vi "Intake Controller.vi"(8 "error in":errorcluster) -> ()   [LabVIEW 2017]
doc: "This VI executes continuously carrying out the current operation and responding to updates or new operations. It will often contain the timing or control code that is difficult to place directly in TeleOp. This VI generally opens all sensors and motors and isolates the rest of the robot code from knowing how the operations are carried out."
uses:
  <vilib>/Rock Robotics/WPI/Framework/Completion Status.ctl
  Intake Setpoints.ctl
  Intake Operations.ctl
  <vilib>/Rock Robotics/SystemInterfaces/DIO/FPGA_DIOPWMChannel.ctl
  <vilib>/Rock Robotics/WPI/RobotDrive/WPI_RobotDriveOpen2MotorWithSPARK.vi
  <vilib>/Rock Robotics/Network Tables/NT Write Boolean.vi
  Framework/Robot Global Data.vi
panel:
  in  "Interactive Values":T1
  out "Current\nCmd":string="Started at  12:56:38.436\nDefault: Reserve,  S 0.0, D 0.000000"
  in  "Buttons":cluster{"Execute Cmd":bool, "Abort Cmd":bool}
  out "Command Timing":cluster{"Start Time (ms)":u32, "Iterations":i32}={"Start Time (ms)"=8116528, "Iterations"=0}
  out "Status":T3
  # "Tip: It may be helpful to observe inputs and sensor values.\nYou may also want to display tuning or debugging controls."
  # "Interactive Command: You may fill in the settings for a command\nand schedule it with the Execute button. You can observe and abort\nany command while fine tuning the code for the controller."
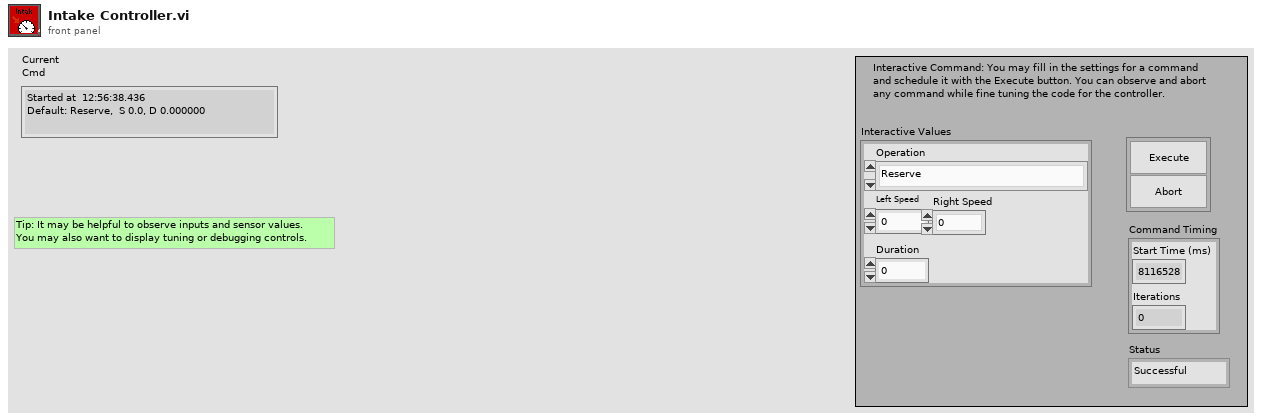
[diagram p1: front panel]
types:
  T1 = typedef "Intake Setpoints.ctl" = cluster{"Operation":T2, "Left Speed":dbl, "Duration":dbl, "Right Speed":dbl}
  T2 = typedef "Intake Operations.ctl" = enum16{"Reserve", "Read Current", "Immediate", "Intake for Duration", "Intake Until Cube"}
  T3 = typedef "Completion Status.ctl" = enum16{"Successful", "Aborted", "Incomplete"}
  T4 = typedef "FPGA_DIOPWMChannel.ctl" = enum8{"PWM 0", "PWM 1", "PWM 2", "PWM 3", "PWM 4", "PWM 5", "PWM 6", "PWM 7", "PWM 8", "PWM 9", "PWM MXP 0", "PWM MXP 1", "PWM MXP 2", "PWM MXP 3", "PWM MXP 4", "PWM MXP 5", "PWM MXP 6", "PWM MXP 7", "PWM MXP 8", "PWM MXP 9", "Invalid"}
  T5 = typedef "WPI_RobotDriveDevRef.ctl" = cluster{"DevStatus":errorcluster, "Motors[]":T6[], "Square Inputs":bool, "Max Output":dbl}
  T6 = typedef "WPI_MotorControlDeviceRef.ctl" = cluster{"DeviceStatus":errorcluster, "Type":T7, "PWM":cluster{"PWM Channel":T4, "DeadBand":T8}, "CAN":cluster{"Device Number":u8, "SetOutput VI Ref":variant, "GetOutput VI Ref":variant, "Enable VI Ref":variant, "Disable VI Ref":variant, "Data":variant}, "Invert":bool, "DIO PWM":cluster{"PWM \"Enable\" Channel":T4, "DIOChannel":T9, "PWM Rate":dbl}}
  T7 = typedef "WPI_MotorControlType.ctl" = enum16{"PWM", "CAN", "DIO PWM"}
  T8 = typedef "WPI_PWMDeadband.ctl" = cluster{"Name":string, "maxPositivePwm":i32, "minPositivePwm":i32, "centerPwm":i32, "maxNegativePwm":i32, "minNegativePwm":i32, "angularRange":u16}
  T9 = typedef "FPGA_DIOChannel.ctl" = enum8{"DIO 0", "DIO 1", "DIO 2", "DIO 3", "DIO 4", "DIO 5", "DIO 6", "DIO 7", "DIO 8", "DIO 9", "DIO MXP 0", "DIO MXP 1", "DIO MXP 2", "DIO MXP 3", "DIO MXP 4", "DIO MXP 5", "DIO MXP 6", "DIO MXP 7", "DIO MXP 8", "DIO MXP 9", "DIO MXP 10", "DIO MXP 11", "DIO MXP 12", "DIO MXP 13", "DIO MXP 14", "DIO MXP 15", "SPI Port CS1", "SPI Port CS2", "SPI Port CS3", "SPI Port MISO", "SPI Port MOSI", "Invalid"}
  T10 = typedef "Command Status Info.ctl" = cluster{"Name":string, "Status":T3, "notifier out":T11}
  T11 = typedef "Completion Notifier.ctl" = refnum<notifier>
  T12 = cluster{"Current Command":T1, "Command Timing":cluster{"Start Time (ms)":u32, "Iterations":i32}, "Command Arguments":cluster{"Command Info":T10, "Description":string, "Default Command":T1, "queue out":refnum<queue>, "Subsystem Name":string}}
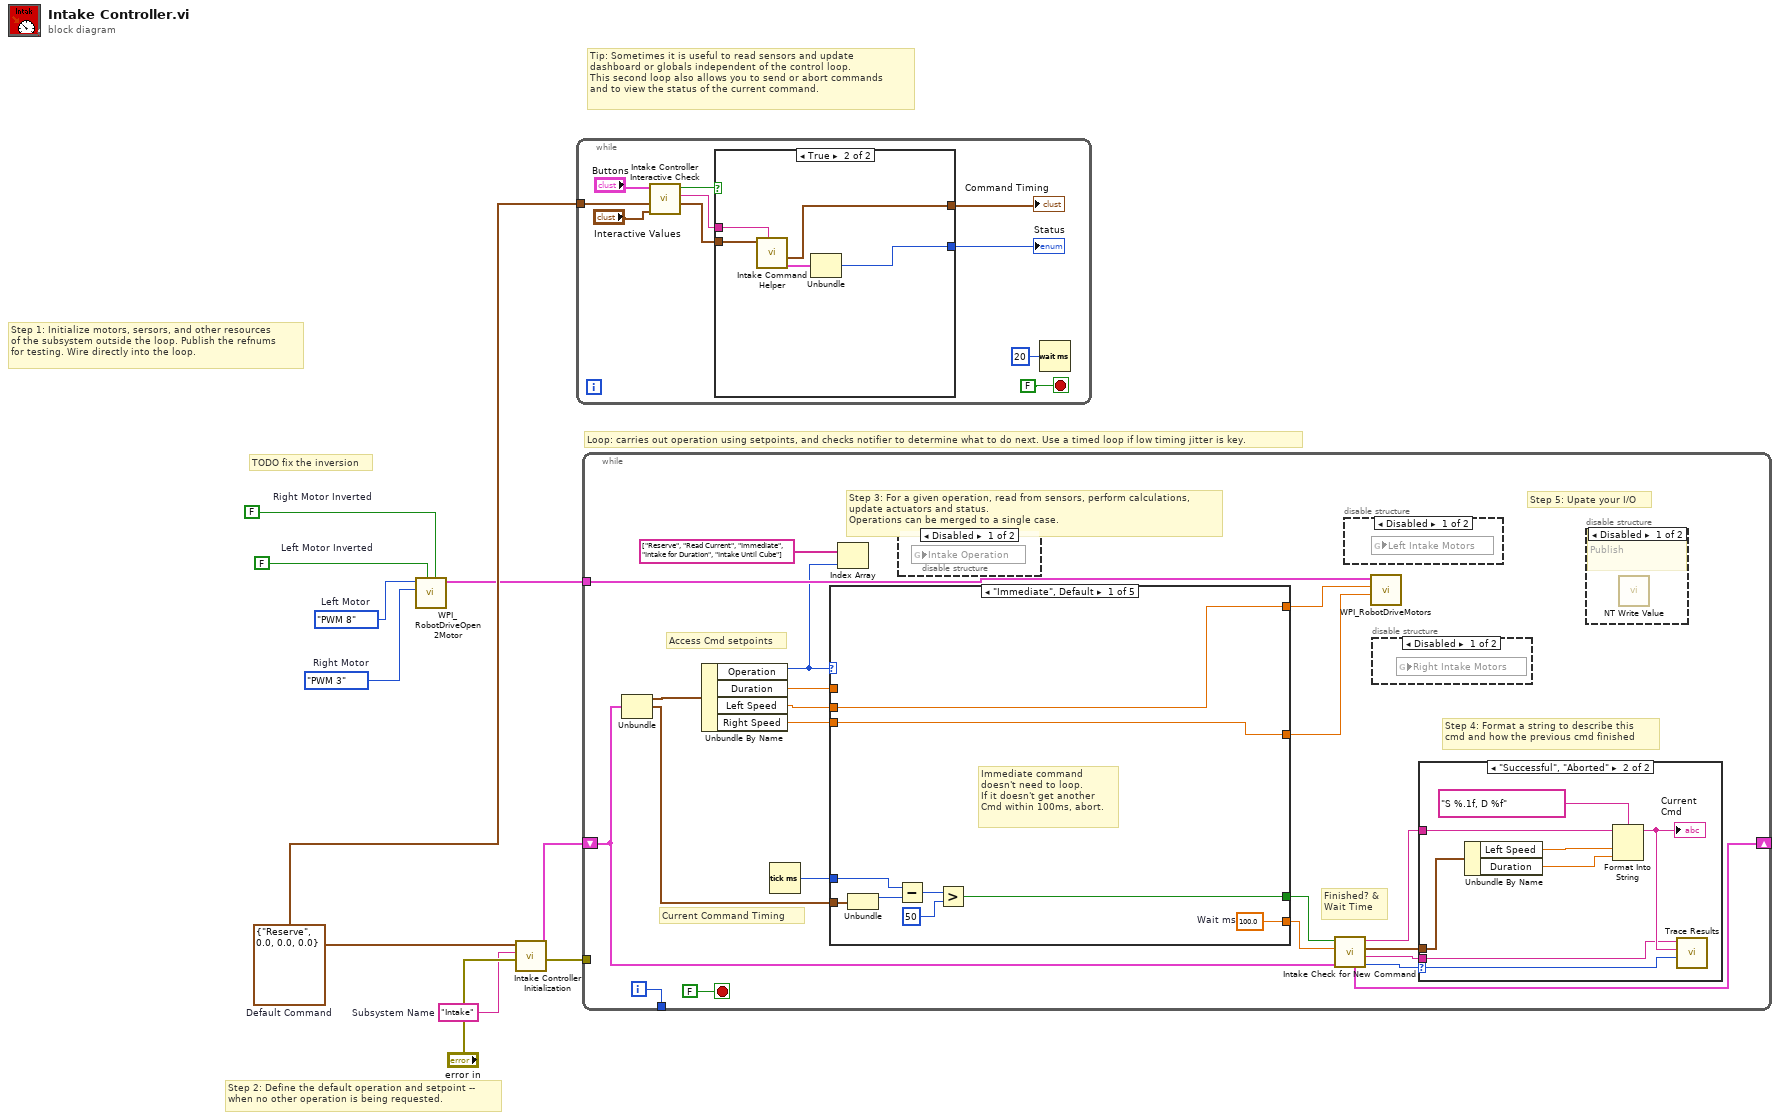
[diagram p0: block diagram]
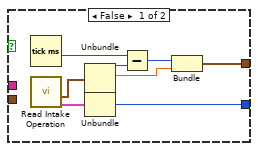
[diagram p2: hidden frame]
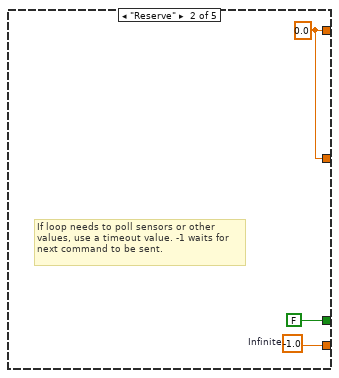
[diagram p6: hidden frame]
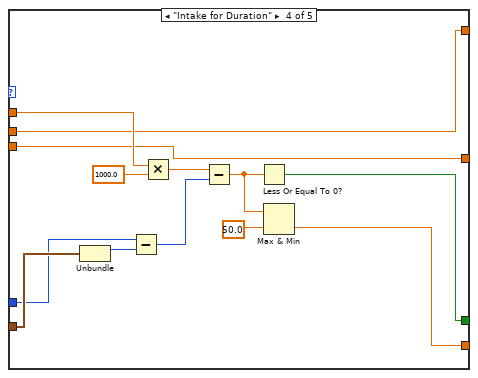
[diagram p8: hidden frame]
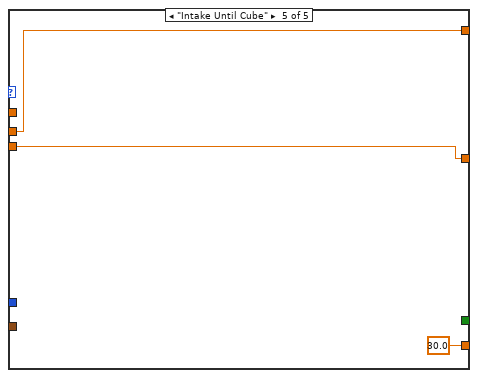
[diagram p9: hidden frame]
diagram:
  w1 = FALSE  # Left Motor Inverted
  w4 = FALSE  # Right Motor Inverted
  w2 = FPGA_DIOPWMChannel."PWM 3"  # Right Motor
  w3 = FPGA_DIOPWMChannel."PWM 8"  # Left Motor
  w6 = T1 {"Operation"=enum."Reserve", "Left Speed"=0.0, "Duration"=0.0, "Right Speed"=0.0}  # Default Command
  w7 = "Intake"  # Subsystem Name
  # "Step 2: Define the default operation and setpoint --\nwhen no other operation is being requested."
  # "TODO fix the inversion"
  # "Tip: Sometimes it is useful to read sensors and update\ndashboard or globals independent of the control loop.\nThis second loop also allows you to send or abort commands\nand to view the status of the current command."
  # "Step 1: Initialize motors, sersors, and other resources\nof the subsystem outside the loop. Publish the refnums\nfor testing. Wire directly into the loop."
  # "Loop: carries out operation using setpoints, and checks notifier to determine what to do next. Use a timed loop if low timing jitter is key."
  n1 = call-poly <vilib>:"WPI_RobotDriveOpen2Motor.vi"("Right Motor Inverted"=w4, "Left Motor Inverted"=w1, "Right Motor"=w2, "Left Motor"=w3) -> ("RobotDriveDevRef"=w5:T5)  [unwired: 6 in, 1 out]
  n2 = call "Intake Controller Initialization.vi"("Subsystem Name"=w7, "Default Command"=w6) -> ("Current Command"=w8:T12)  [unwired: 9 in]
  n3 = while {
    tunnel: w6 -> [w16]
    stop <- FALSE stop-if-true
    n4 = call "Intake Controller Interactive Check.vi"("Interactive Command in"="Interactive Values", "Default Command"=w16, "Buttons"="Buttons") -> ("Interactive Command out"=w13:T1, "Trace String"=w14:string, "Schedule"=w15:bool)  [unwired: 6 in]
    n5 = case shown="True" w15 {
      tunnel: [w27 w32] -> w12
      tunnel: w13 -> [_ w30]
      tunnel: [w23 w28] -> w11
      tunnel: w14 -> [_ w31]
      frame False {
        n6 = Tick Count (ms)() -> (millisecond timer value=w22:u32)
        n7 = call "Read Intake Operation.vi"() -> ("Command Info"=w20:T10, "SubSystem Data"=w21:T1)  [unwired: 9 in, 1 out]
        n8 = Unbundle(w21) -> ("Operation"=w26:T2, "Left Speed"=w24:dbl)  [unwired: 2 out]
        n9 = Unbundle(w20) -> ("Status"=w27:T3)  [unwired: 2 out]
        n10 = Subtract(x=w22, y=w26) -> (x-y=w25:u32)
        n11 = Bundle(w25, "Left Speed"=w24) -> (w23:cluster{u32, "Left Speed":dbl})  [unwired: 1 in]
      }
      frame True {
        n12 = call "Intake Command Helper.vi"("Description"=w31, "SubSystem Data"=w30) -> ("Command Info Out"=w29:T10, "Command Timing"=w28:cluster{"Start Time (ms)":u32, "Iterations":i32})  [unwired: 7 in, 1 out]
        n13 = Unbundle(w29) -> ("Status"=w32:T3)  [unwired: 2 out]
      }
    }
    "Status" <- w12
    "Command Timing" <- w11
    n14 = Wait (ms)(milliseconds to wait=u32 20) -> ()  [unwired: 1 out]
  }
  n15 = while {
    shift-right: [w46] -> _
    shift-left: w8 -> [w39]
    tunnel: [w52] -> _
    tunnel: "error in" -> [_]
    tunnel: w5 -> [w38]
    i -> [w52]
    stop <- FALSE stop-if-true
    # "Step 5: Upate your I/O"
    # "Step 4: Format a string to describe this\ncmd and how the previous cmd finished"
    # "Current Command Timing"
    # "Access Cmd setpoints"
    # "Finished? &\nWait Time"
    # "Step 3: For a given operation, read from sensors, perform calculations,\nupdate actuators and status.\nOperations can be merged to a single case."
    n16 = Unbundle(w39) -> ("Current Command"=w51:T1, "Command Timing"=w48:cluster{"Start Time (ms)":u32, "Iterations":i32})  [unwired: 1 out]
    n17 = Unbundle By Name(w51) -> ("Operation"=w37:T2, "Duration"=w50:dbl, "Left Speed"=w47:dbl, "Right Speed"=w35:dbl)
    n18 = Tick Count (ms)() -> (millisecond timer value=w49:u32)
    n19 = case shown="\"Immediate\", Default" w37 {
      tunnel: [w62 w65 _ w69 30.0 ("Infinite")] -> w44
      tunnel: [w56 FALSE ("ignore previous (F)") _ w70 _] -> w45
      tunnel: w48 -> [w58 _ _ w68 _]
      tunnel: w50 -> [_ _ _ w72 _]
      tunnel: w49 -> [w57 _ _ w67 _]
      tunnel: w47 -> [w55 _ _ w71 w81]
      tunnel: [w55 w63 _ w71 w81] -> w34
      tunnel: [w54 w63 _ w66 w79] -> w33
      tunnel: w35 -> [w54 _ _ w66 w79]
      frame "Immediate", Default {
        w62 = 100.0  # Wait ms
        # "Immediate command\ndoesn't need to loop.\nIf it doesn't get another\nCmd within 100ms, abort."
        n20 = Unbundle(w58) -> ("Start Time (ms)"=w61:u32)  [unwired: 1 out]
        n21 = Subtract(x=w57, y=w61) -> (x-y=w60:u32)
        n22 = Greater?(x=w60, y=u8 50 ("Left Motor")) -> (0:w56:bool)
      }
      frame "Reserve" {
        w63 = 0.0 ("Speed")
        w65 = -1.0  # Infinite
        # "If loop needs to poll sensors or other\nvalues, use a timeout value. -1 waits for\nnext command to be sent."
      }
      frame "Read Current" {
      }
      frame "Intake for Duration" {
        n23 = Unbundle(w68) -> ("Start Time (ms)"=w75:u32)  [unwired: 1 out]
        n24 = Subtract(x=w67, y=w75) -> (x-y=w78:u32)
        n25 = Multiply(x=w72, y=1000.0) -> (x*y=w77:dbl)
        n26 = Subtract(x=w77, y=w78) -> (x-y=w74:dbl)
        n27 = Less Or Equal To 0?(x=w74) -> (x <= 0?=w70:bool)
        n28 = Max & Min(x=w74, y=50.0) -> (min(x,y)=w69:dbl)  [unwired: 1 out]
      }
      frame "Intake Until Cube" {
      }
    }
    n29 = Index Array(array=string[] ["Reserve", "Read Current", "Immediate", "Intake for Duration", "Intake Until Cube"] ("Strings []"), index=w37) -> ()  [unwired: 1 out]
    n30 = disable-structure shown="Disabled" {
      frame Disabled {
        n31 = global read "Robot Global Data.vi" "Intake Operation"() -> ()  [unwired: 1 in]
      }
      frame Enabled {
      }
    }
    n32 = call "Intake Check for New Command.vi"("Current Command"=w39, "Wait time (ms)"=w44, "Finished?"=w45) -> ("Completion"=w40:T3, "Subsystem Name"=w41:string, "Current Command"=w42:T1, "Initial Trace String"=w43:string, "NextCommand"=w46:T12)  [unwired: 4 in]
    n33 = disable-structure shown="Disabled" {
      frame Disabled {
        n34 = global read "Robot Global Data.vi" "Left Intake Motors"() -> ()  [unwired: 1 in]
      }
      frame Enabled {
      }
    }
    n35 = call <vilib>:"WPI_RobotDriveMotors.vi"("RightSpeed"=w33, "LeftSpeed"=w34, "RobotDriveDevRef"=w38) -> ()  [unwired: 1 in, 8 out]
    n36 = disable-structure shown="Disabled" {
      frame Disabled {
        n37 = global read "Robot Global Data.vi" "Right Intake Motors"() -> ()  [unwired: 1 in]
      }
      frame Enabled {
      }
    }
    n38 = case shown="\"Successful\", \"Aborted\"" w40 {
      selector: w40 -> [_ w89]
      tunnel: w43 -> [_ w85]
      tunnel: w42 -> [_ w86]
      tunnel: w41 -> [_ w82]
      frame "Incomplete", Default {
        # "Continuing current command"
      }
      frame "Successful", "Aborted" {
        # "Report and setup for next command"
        n39 = Unbundle By Name(w86) -> ("Left Speed"=w88:dbl, "Duration"=w83:dbl)
        n40 = Format Into String(format string="S %.1f, D %f", initial string=w85, w88, w83) -> (resulting string=w84:string)  [unwired: 1 in, 1 out]
        "Current\nCmd" <- w84
        n41 = call <vilib>:"Trace Results.vi"("Status of previous command"=w89, "Description"=w84, "Subsystem"=w82) -> ()  [unwired: 9 in]
      }
    }
    n42 = disable-structure shown="Disabled" {
      frame Disabled {
        # "Publish"
        n43 = call-poly <vilib>:"NT Write Value.vi"() -> ()  [unwired: 11 in, 1 out]
      }
      frame Enabled {
      }
    }
  }
